vi "TCPinfo.vi"() -> ()   [LabVIEW 2012, in "AccelNET.lvlib" / "Global_Variables.lvlib"]
uses:
  Global_Variables.lvlib
  TCP.lvclass
panel:
  in  "AccelNET.lvlib:TCP.lvclass":refnum<class "TCP.lvclass">
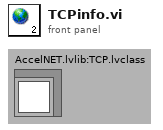
[diagram p1: front panel]
diagram:
